vi "Check If Table Exists.vi"(8 "error in":errorcluster, 10 "Table Name":string, 11 "orm in":refnum<class "LV-ORM.lvclass">) -> (0 "error out":errorcluster, 2 "index of element":i32, 3 "orm out":refnum<class "LV-ORM.lvclass">, 5 "table exists?":bool)   [LabVIEW 2018, in "LV-ORM.lvclass"]
uses:
  LV-ORM.lvclass
  LV-ORM.lvclass/LV-ORM.ctl
  <vilib>/addons/database/NI_Database_API.lvlib
panel:
  out "tables":string[](array[string])
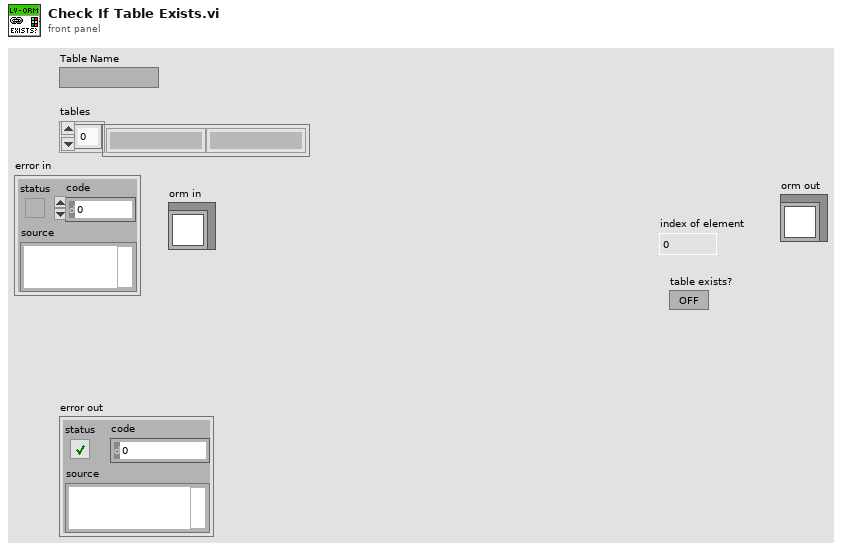
[diagram p1: front panel]
types:
  T1 = typedef "NI_Database_API.lvlib/Conn ObjectReference.ctl" = refnum<k1>
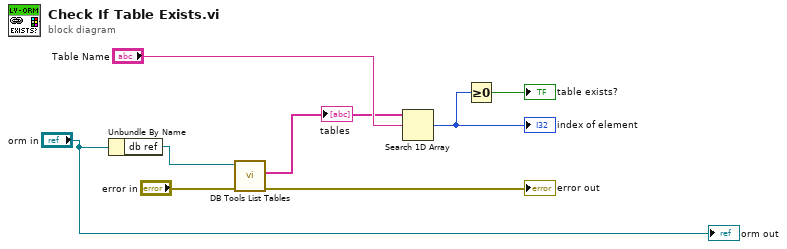
[diagram p0: block diagram]
diagram:
  n1 = Unbundle By Name("orm in") -> ("db ref"=w2:T1)
  n2 = call <vilib>:"DB Tools List Tables.vi"("error in (no error)"="error in", "connection reference"=w2) -> ("error out"=→"error out":errorcluster, "tables"=w5:string[])  [unwired: 3 in, 1 out]
  "tables" <- w5
  n3 = Search 1D Array(1D array=w5, element="Table Name") -> (index of element=w6:i32)  [unwired: 1 in]
  "index of element" <- w6
  n4 = Greater Or Equal To 0?(x=w6) -> (x >= 0?=→"table exists?":bool)
  "orm out" <- "orm in"
